vi "Write Elements of TemporaryPath.vi"(8 "error in (no error)":errorcluster, 10 "Paths":path[](array[path]), 11 "Folder_Mgmt":refnum<class "Folder_Mgmt.lvclass">) -> (0 "error out":errorcluster, 3 "Folder_Mgmt 2":refnum<class "Folder_Mgmt.lvclass">)   [LabVIEW 2016, in "Folder_Mgmt.lvclass"]
uses:
  Folder_Mgmt.lvclass
  Folder_Mgmt.lvclass/Folder_Mgmt.ctl
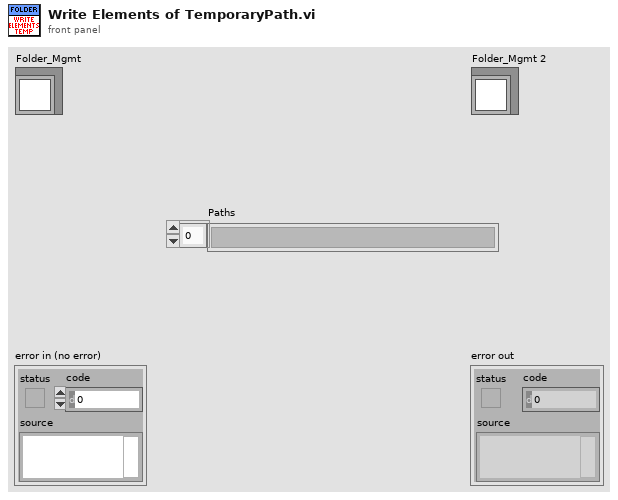
[diagram p1: front panel]
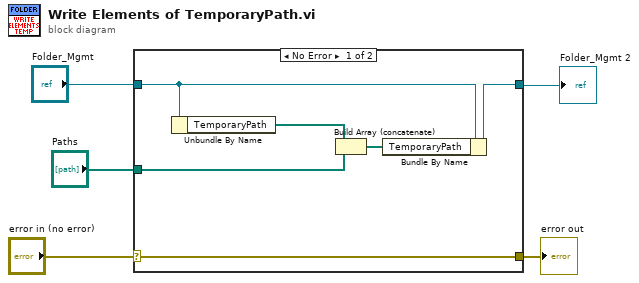
[diagram p0: block diagram]
diagram:
  n1 = case shown="No Error" "error in (no error)" {
    selector: "error in (no error)" -> [w11 w12]
    tunnel: [w11 w12] -> w4
    tunnel: [w9 w13] -> w1
    tunnel: "Folder_Mgmt" -> [w8 w13]
    tunnel: "Paths" -> [w10 _]
    frame No Error {
      n2 = Unbundle By Name(w8) -> ("TemporaryPath"=w6:path[])
      n3 = Build Array (concatenate)(w6, w10) -> (w7:path[])
      n4 = Bundle By Name(cluster=w8, "TemporaryPath"=w7) -> (w9:refnum<class "Folder_Mgmt.lvclass">)
    }
    frame Error {
    }
  }
  "error out" <- w4
  "Folder_Mgmt 2" <- w1
